vi "set_sample_dwell_time.vi"(8 "error in (no error)":errorcluster, 10 "sample dwell time":dbl[unit], 11 "GenericWriteSignals.lvclass in":refnum<class "SignalWriterDL101123SoundCard.lvclass">) -> (0 "error out":errorcluster, 3 "GenericWriteSignals.lvclass out":refnum<class "SignalWriterDL101123SoundCard.lvclass">)   [LabVIEW 2010, in "SignalWriterDL101123SoundCard.lvclass"]
uses:
  SignalWriterDL101123SoundCard.lvclass
  GenericSignalWriter/GenericSignalWriter/GenericSignalWriter.lvclass
  SignalWriterDL101123SoundCard.lvclass/SignalWriterDL101123SoundCard.ctl
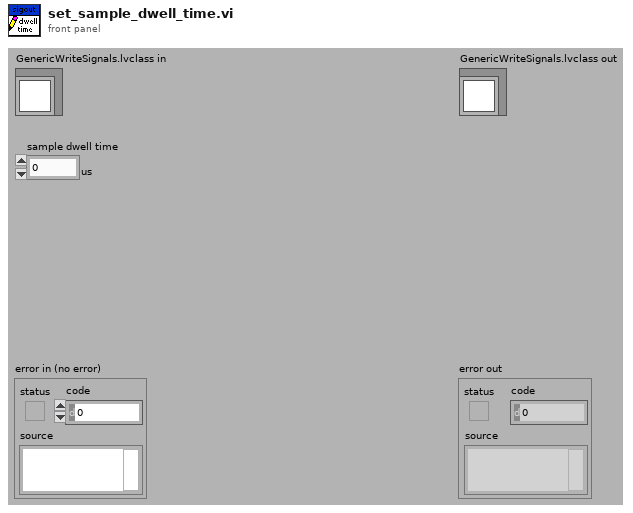
[diagram p1: front panel]
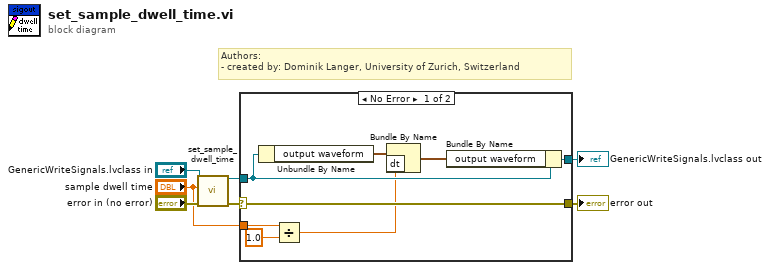
[diagram p0: block diagram]
diagram:
  # "Authors: \n- created by: Dominik Langer, University of Zurich, Switzerland"
  n1 = call-parent "set_sample_dwell_time.vi"("error in (no error)"="error in (no error)", "sample dwell time"="sample dwell time", "GenericWriteSignals.lvclass in"="GenericWriteSignals.lvclass in") -> ("error out"=w4:errorcluster, "GenericWriteSignals.lvclass out"=w5:refnum<class "SignalWriterDL101123SoundCard.lvclass">)  [unwired: 7 in]
  n2 = case shown="No Error" w4 {
    selector: w4 -> [w14 w17]
    tunnel: w5 -> [w13 w16]
    tunnel: [w14 w17] -> w3
    tunnel: "sample dwell time" -> [w9 _]
    tunnel: [w11 w16] -> w1
    frame No Error {
      n3 = Unbundle By Name(w13) -> ("output waveform"=w15:waveform(dbl))
      n4 = Divide(x=w9, y=dbl[unit] 1.0) -> (x/y=w8:dbl)
      n5 = Bundle By Name(cluster=w15, "dt"=w8) -> (w12:waveform(dbl))
      n6 = Bundle By Name(cluster=w13, "output waveform"=w12) -> (w11:refnum<class "SignalWriterDL101123SoundCard.lvclass">)
    }
    frame Error {
    }
  }
  "error out" <- w3
  "GenericWriteSignals.lvclass out" <- w1
